vi "Change Copy LLB to NI VeriStand.vi"(8 "error in (no error)":errorcluster, 9 "CD Template":refnum<class "NIVS_CD Template.lvclass">, 10 "Copy .LLB to ... path":path, 11 "CD Name":string) -> (0 "error out":errorcluster)   [LabVIEW 2020, in "NIVS_Consolidated_CDW_MetaDataObj.lvclass"]
doc: "Change the block diagram of \"Copy .LLB to NI VeriStand dir\" accoding to the custom device name and the execution mode."
uses:
  NIVS_Consolidated_CDW_MetaDataObj.lvclass
  Template Classes/NIVS_CD Template/NIVS_CD Template.lvclass
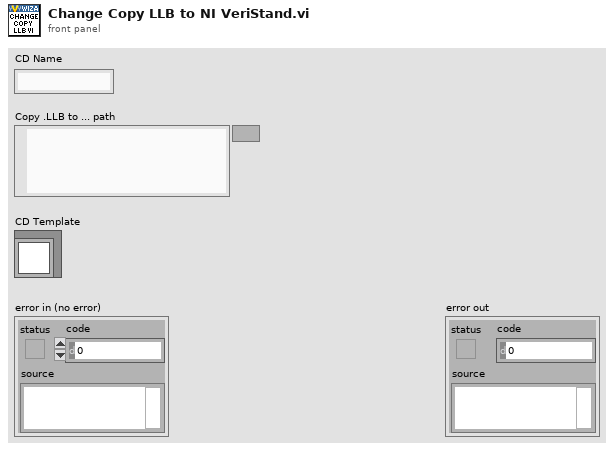
[diagram p1: front panel]
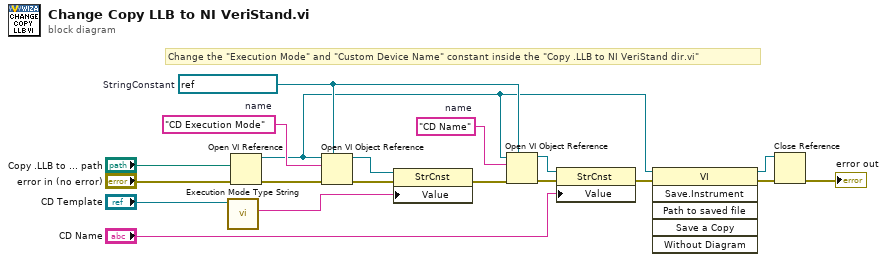
[diagram p0: block diagram]
diagram:
  w10 = "CD Name"  # name
  w15 = "CD Execution Mode"  # name
  w11 = refnum<vi> refnum  # StringConstant
  # "Change the \"Execution Mode\" and \"Custom Device Name\" constant inside the \"Copy .LLB to NI VeriStand dir.vi\""
  n1 = call-dynamic "Execution Mode Type String.vi"("CD Template"="CD Template") -> ("Execution Mode Type String"=w1:string)  [unwired: 10 in]
  n2 = Open VI Reference(vi path="Copy .LLB to ... path", error in (no error)="error in (no error)") -> (vi reference=w4:refnum<vi>, error out=w3:errorcluster)  [unwired: 4 in]
  n3 = Open VI Object Reference(7:w11, 8:w3, 10:w15, 11:w4) -> (0:w14:errorcluster, 3:w12:refnum<vi>)
  n4 = property class="StrCnst"(reference=w12, error in=w14, "Value"=w1) -> (error out=w13:errorcluster)  [unwired: 1 out]
  n5 = Open VI Object Reference(7:w11, 8:w13, 10:w10, 11:w4) -> (0:w9:errorcluster, 3:w8:refnum<vi>)
  n6 = property class="StrCnst"(reference=w8, error in=w9, "Value"="CD Name") -> (error out=w5:errorcluster)  [unwired: 1 out]
  n7 = invoke class="VI" method="Save.Instrument"(reference=w4, error in=w5) -> (reference out=w7:refnum<vi>, error out=w6:errorcluster)  [unwired: 4 in, 4 out]
  n8 = Close Reference(reference=w7, error in (no error)=w6) -> (error out=→"error out":errorcluster)
